vi "Create PathArrayMsg.vi"(8 "error in (no error)":errorcluster, 10 "Message Data":path[](array[path]), 11 "Message Name":string) -> (0 "error out":errorcluster, 3 "PathArrayMsg out":refnum<class "PathArrayMsg.lvclass">)   [LabVIEW 2018, in "LapDog.Messaging.v3.NativeArrays.lvlib" / "PathArrayMsg.lvclass"]
doc: "Returns a PathArrayMsg object with the given name.\n\nThis method executes regardless of the error in state."
uses:
  PathArrayMsg.lvclass
  T:/git/LapDog.Messaging/src/LapDog.Messaging/Message/Message.lvclass
  PathArrayMsg.lvclass/PathArrayMsg.ctl
  LapDog.Messaging/Message/Message.lvclass
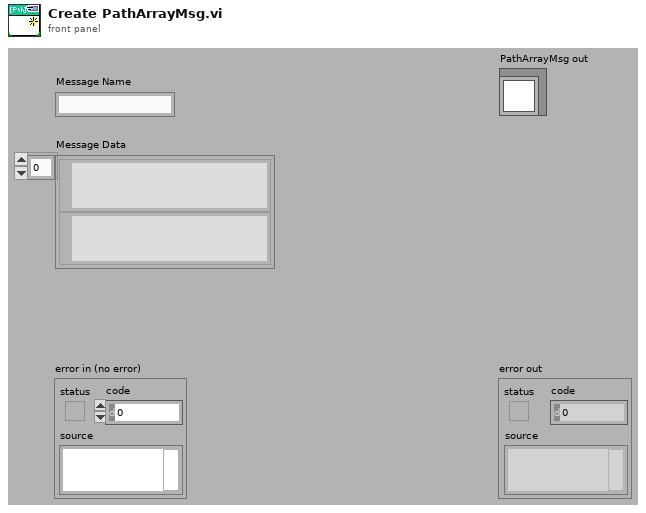
[diagram p1: front panel]
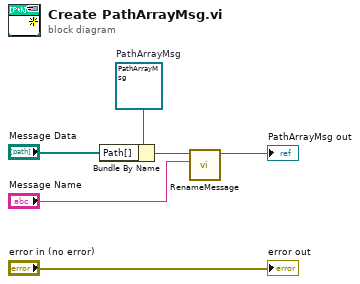
[diagram p0: block diagram]
diagram:
  w1 = refnum<class "PathArrayMsg.lvclass"> refnum  # PathArrayMsg
  n1 = Bundle By Name(cluster=w1, "Path[]"="Message Data") -> (w4:refnum<class "PathArrayMsg.lvclass">)
  n2 = call "RenameMessage.vi"("Message Name"="Message Name", "Message in"=w4) -> ("Message out"=→"PathArrayMsg out":refnum<class "PathArrayMsg.lvclass">)  [unwired: 8 in, 1 out]
  "error out" <- "error in (no error)"
